vi "Hardware Out - NI 9752-1 (AD Combo).vi"(11 "FPGA Ref":T1) -> ()   [LabVIEW 2015, in "ECS-RT.lvlib"]
uses:
  ECS-RT.lvlib
  Typedefs/FPGA Refs/Generic FPGA Ref.ctl
  <vilib>/Utility/error.llb/Error Cluster From Error Code.vi
  <vilib>/rvi/errors/niLvFpgaAdjustHostInterfaceError.vi
  <vilib>/rvi/interface/nirviReadWriteControl/nirviReadWriteControl.xnode
  <vilib>/rvi/interface/Simulation/niFpgaSimulationCallBeginRW.vi
  NiFpgaLv.dll
  ECS-Shared.lvlib
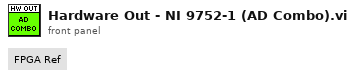
[diagram p1: front panel]
types:
  T1 = typedef "ECS-Shared.lvlib/Generic FPGA Ref.ctl" = refnum<k20>
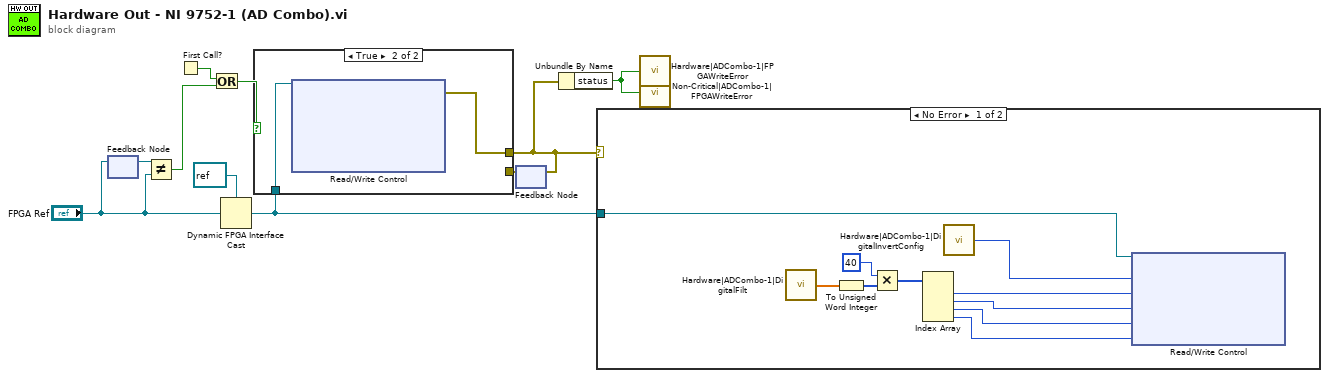
[diagram p0: block diagram]
diagram:
  n1 = feedback #1() -> (w9:T1)  [unwired: 1 in]
  n2 = feedback-in #1("FPGA Ref") -> ()
  n3 = Not Equal?(x=w9, y="FPGA Ref") -> (x != y?=w10:bool)
  n4 = First Call?() -> (First Call?: T/F=w8:bool)
  n5 = Or(x=w8, y=w10) -> (x .or. y?=w7:bool)
  n6 = Dynamic FPGA Interface Cast(Session In=refnum<k20> refnum ("NI 9757 (ADCombo)"), Type="FPGA Ref") -> (Session Out=w3:refnum<k20>)
  n7 = feedback #2() -> (w6:errorcluster)  [unwired: 1 in]
  n8 = case shown="True" w7 {
    tunnel: [w11 w12] -> w2
    tunnel: w6 -> [w11 _]
    tunnel: w3 -> [_ w13]
    frame False {
    }
    frame True {
      n9 = xnode "Read/Write Control"("FPGA VI Reference In"=w13) -> ("error out"=w12:errorcluster)  [unwired: 6 in, 1 out]
    }
  }
  n10 = feedback-in #2(w2) -> ()
  n11 = Unbundle By Name(w2) -> ("status"=w1:bool)
  n12 = case shown="No Error" w2 {
    tunnel: w3 -> [w14 _]
    frame No Error {
      n13 = call "Hardware|ADCombo-1|DigitalFilt"() -> ("Value"=w23:sgl[])
      n14 = To Unsigned Word Integer(number=w23) -> (unsigned 16bit integer=w22:u16[])
      n15 = Multiply(x=u16 40 ("y"), y=w22) -> (x*y=w21:u16[])
      n16 = Index Array(array=w21) -> (element #1=w20:u16, element #2=w19:u16, element #3=w18:u16, element #4=w17:u16)  [unwired: 4 in]
      n17 = call "Hardware|ADCombo-1|DigitalInvertConfig"() -> ("Value"=w15:u32)
      n18 = xnode "Read/Write Control"("FPGA VI Reference In"=w14, "ADCombo-1.VRHallInvert"=w15, "ADCombo-1.VR1.Filt"=w20, "ADCombo-1.VR2.Filt"=w19, "ADCombo-1.Hall1.Filt"=w18, "ADCombo-1.Hall2.Filt"=w17) -> ()  [unwired: 1 in, 2 out]
    }
    frame Error {
    }
  }
  n19 = call "Hardware|ADCombo-1|FPGAWriteError"("Value"=w1) -> ()
  n20 = call "Non-Critical|ADCombo-1|FPGAWriteError"("Fault"=w1) -> ()  [unwired: 2 in]
